vi "Get DBL.vi"(8 "error in (no error)":errorcluster, 9 "Data Type (default value)":dbl, 10 "Offset":i32, 11 "JSON":string) -> (0 "error out":errorcluster, 1 "Number":dbl format="%.2f", 2 "Offset past match":i32)   [LabVIEW 2020, in "JSONtext.lvlib"]
uses:
  <vilib>/JDP Science/JSONtext/JSONtext.lvlib
  <vilib>/JDP Science/JSONtext/String Subset.vi
  <vilib>/JDP Science/JSONtext/Parsing/Advance past Number.vi
  <vilib>/JDP Science/JSONtext/Parsing/Parsing Error in converting to LabVIEW type.vi
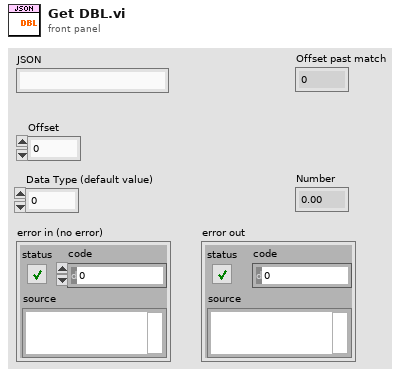
[diagram p1: front panel]
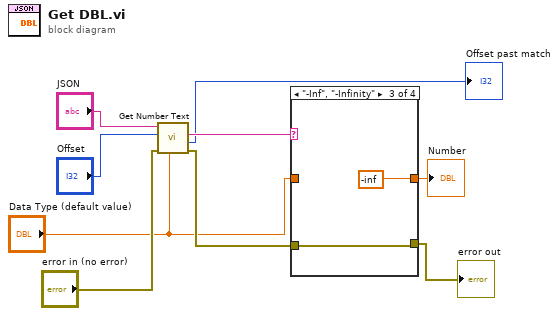
[diagram p0: block diagram]
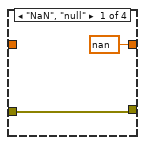
[diagram p2: hidden frame]
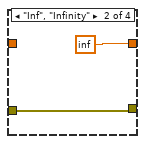
[diagram p3: hidden frame]
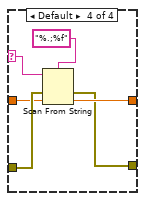
[diagram p4: hidden frame]
diagram:
  n1 = call <vilib>:"Get Number Text.vi"("LV Type"="Data Type (default value)", "error in (no error)"="error in (no error)", "Offset"="Offset", "JSON"="JSON") -> ("error out"=w6:errorcluster, "Offset past match"=→"Offset past match":i32, "Number Text"=w4:string)  [unwired: 4 in, 1 out]
  n2 = case shown="\"-Inf\", \"-Infinity\"" w4 {
    selector: w4 -> [_ _ _ w17]
    tunnel: [nan ("default value 1") inf ("default value 1") -inf ("default value 1") w21] -> w3
    tunnel: w6 -> [w11 w12 w14 w20]
    tunnel: [w11 w12 w14 w19] -> w5
    tunnel: "Data Type (default value)" -> [_ _ _ w18]
    frame "NaN", "null" {
    }
    frame "Inf", "Infinity" {
    }
    frame "-Inf", "-Infinity" {
    }
    frame Default {
      n3 = Scan From String(format string="%.;%f", input string=w17, error in=w20, default 1=w18) -> (error out=w19:errorcluster, output 1=w21:dbl)  [unwired: 1 in, 2 out]
    }
  }
  "error out" <- w5
  "Number" <- w3
